vi "Test Message Included if Description is Empty.vi"(8 "error in (no error)":errorcluster, 11 "Test Assertion Results in":refnum<class "Assertion Result Test.lvclass">) -> (0 "error out":errorcluster, 3 "Test Assertion Results out":refnum<class "Assertion Result Test.lvclass">)   [LabVIEW 2020, in "LUnit Tests.lvlib" / "Assertion Result Test.lvclass"]
uses:
  Assertion Result Test.lvclass
  Test Dummys/Test Case Test Double/Test Case Test Double.lvclass
  f7ba8c47-45cd-4aa1-a224-e1b0f819248a.vi
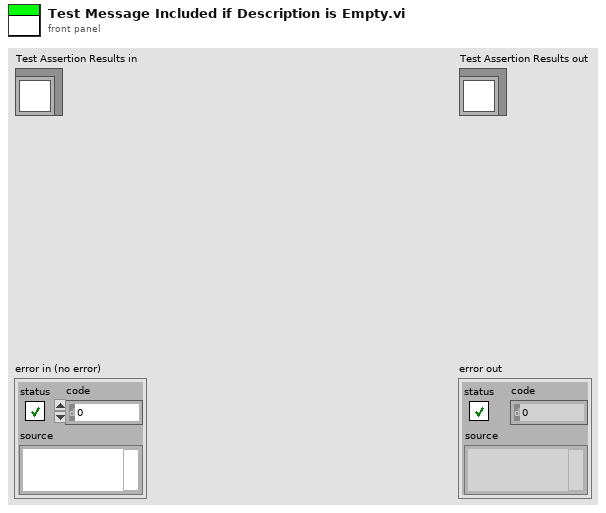
[diagram p1: front panel]
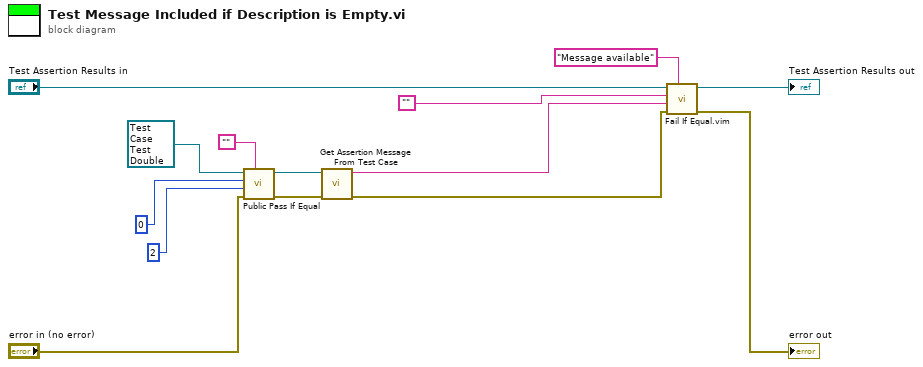
[diagram p0: block diagram]
diagram:
  n1 = call "Public Pass If Equal.vi"("Description"="", "error in (no error)"="error in (no error)", "Actual"=2, "Expected"=0, "Test Case Test Double in"=refnum<class "Test Case Test Double.lvclass"> refnum ("Test Case Test Double.lvclass")) -> ("error out"=w11:errorcluster, "Test Case Test Double out"=w12:refnum<class "Test Case Test Double.lvclass">)  [unwired: 5 in]
  n2 = call "Get Assertion Message From Test Case.vi"("error in (no error)"=w11, "Test Case Test Double in"=w12) -> ("error out"=w6:errorcluster, "Message"=w5:string)  [unwired: 8 in]
  n3 = call "Fail If Equal.vim"("Description"="Message available", "error in (no error)"=w6, "Actual"=w5, "Expected"="" ("Description"), "LUnit Test Case In"="Test Assertion Results in") -> ("error out"=→"error out":errorcluster, "LUnit Test Case Out"=→"Test Assertion Results out":refnum<class "Assertion Result Test.lvclass">)  [unwired: 5 in]
